vi "运维调试_采配水.vi"() -> ()   [LabVIEW 2016, in "PLC.lvlib"]
uses:
  PLC.lvlib
  control/switch.ctl
  <vilib>/Plasmionique/MB Master/MB_Master/MB_Master.lvclass
  <vilib>/Utility/miscctls.llb/LVPointTypeDef.ctl
  <vilib>/Plasmionique/MB Master/MB_Master_Serial/MB_Master_Serial.lvclass
  D:/Program Files (x86)/National Instruments/LabVIEW 2016/vi.lib/Plasmionique/MB Master/MB_Master/MB_Master.lvclass
  <vilib>/Instr/_visa.llb/VISA Configure Serial Port (Instr).vi
  <vilib>/NI/Modbus Library/API/Wrapper/Create TCP Slave.vi
  <vilib>/NI/Modbus Library/API/slave/Modbus Slave.lvclass
  <vilib>/Plasmionique/MB Master/MB Master.lvlib
  <vilib>/ptbypt/NI_PtbyPt.lvlib
  <vilib>/NI/Modbus Library/API/Wrapper/API Main.lvlib
panel:
  in  "63μm反冲洗阀":bool
  out "R34":u16
  in  "Y21":T1
  out "供水压力":dbl format="%.4f"
  out "R44":u16
  in  "Y31":T1
  out "R111":i16 caption="三级水样池润洗时间"
  in  "三级过滤系统":bool
  out "R110":i16 caption="集气时间"
  out "R104":i16 caption="三级润洗时间"
  out "R103":i16 caption="二级润洗时间"
  out "R107":i16 caption="进气时间"
  out "R43":u16
  in  "Y30":T1
  out "Registers":u16[](array[numeric])
  out "R124":i16 caption="加标回收配水时间"
  out "R42":i16
  in  "Y29":T1
  in  "更新程序":T1
  out "R122":i16 caption="二级自来水清洗时间"
  out "R121":i16 caption="一级自来水清洗时间"
  out "R120":i16 caption="过滤自来水清洗时间"
  out "清洗次数":u16
  out "当前启动泵号":u16(ring) items=["1号泵", "2号泵"]
  out "R116":i16 caption="储水时间"
  in  "R113":u16(ring) caption="水箱储水水体" items=["自来水", "水样"]
  out "R112":i16 caption="二级水样池进样超时"
  out "R31":u16
  out "R30":u16
  out "R29":u16
  out "R28":u16
  out "R27":u16
  out "R26":u16
  out "R25":u16
  out "R24":u16
  out "R23":u16
  out "R22":u16
  out "R21":u16
  out "R20":u16
  out "R19":u16
  out "R18":u16
  out "R17":u16
  out "R16":u16
  out "R15":u16
  out "R14":u16
  out "R13":u16
  out "配水压力":dbl format="%.4f"
  in  "Y18":T1
  in  "Y17":T1
  in  "Y14":T1
  in  "Y13":T1
  in  "Y1":T1
  in  "Y0":T1
  in  "Y12":T1
  in  "Y11":T1
  in  "Y10":T1
  in  "Y9":T1
  in  "Y8":T1
  in  "Y7":T1
  out "X2":bool caption="X1"
  out "采配水版本号":string
  out "R117":i16 caption="清洗频次设定"
  out "通讯故障":bool
  in  "R100":u16(ring) caption="采水泵工作模式" items=["泵1单泵单管路", "泵2单泵单管路", "潜水泵双泵双管路", "自吸泵双泵双管路"]
  out "X10":bool caption="氨氮水样池液位开关SL3"
  out "X9":bool caption="泵2过载报警_KM2"
  out "X8":bool caption="泵1过载报警_KM1"
  out "X7":bool caption="断电检测_PA"
  out "X6":bool caption="门禁开关_AS"
  out "X5":bool caption="烟雾检测_SA"
  out "X4":bool caption="浸水检测_WIA"
  out "X3":bool caption="水流开关_FS"
  out "X1":bool
  out "X0":bool caption="采样池液位开关_SL1"
  out "R109":i16 caption="外部反冲洗时间"
  out "集成报警信息":string
  out "R108":i16 caption="进样超时时间"
  out "R106":i16 caption="排液时间"
  out "R105":i16 caption="常规模式配水时间"
  out "R102":i16 caption="沉淀时间"
  out "R101":i16 caption="一级润洗时间"
  out "R2":i16
  out "R1":i16
  out "多列列表框":i32(listbox)
  in  "Y6":T1
  in  "Y5":T1
  in  "Y4":T1
  in  "Y3":T1
  in  "Y2":T1
  in  "Y16":T1
  in  "Y15":T1
  in  "返回":T1
  in  "参数设置":T1
  in  "单步启动":T1
  in  "启动":T1
  in  "停止":T1
  # "s"
  # "流程计时："
  # "s"
  # "单步计时："
  # "MPa"
  # "配水压力："
  # "MPa"
  # "供水压力："
  # "S"
  # "S"
  # "S"
  # "S"
  # "S"
  # "S"
  # "S"
  # "S"
  # "S"
  # "S"
  # "S"
  # "次"
  # "S"
  # "S"
  # "S"
  # "S"
  # "S"
  # "S"
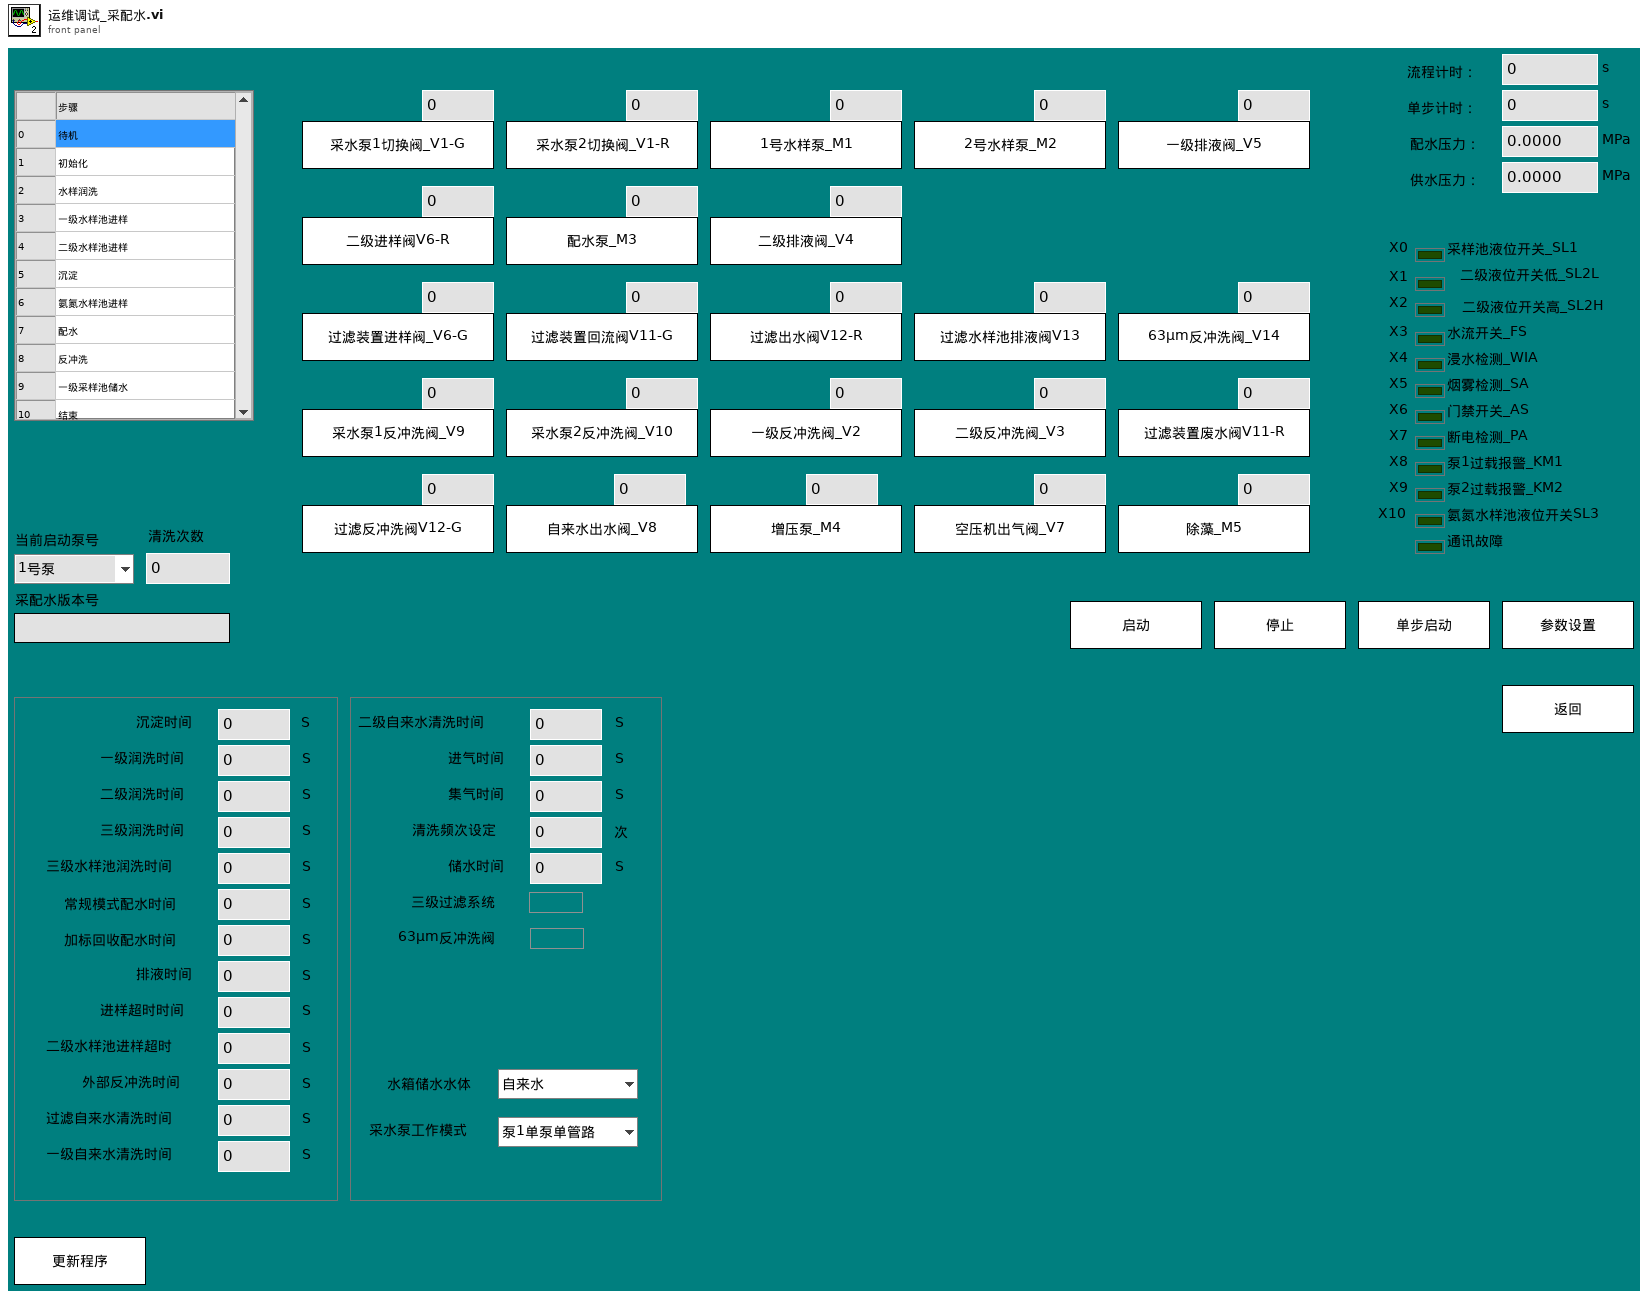
[diagram p1: front panel]
types:
  T1 = typedef "PLC.lvlib/switch.ctl" = bool
  T2 = cluster{"参数启用":cluster{"氨氮":bool, "总磷":bool, "总氮":bool, "多参数":bool, "CODMn":bool, "CODcr":bool, "超标留样":bool}}
  T3 = typedef "LVPointTypeDef.ctl" = cluster{"Horizontal":i16, "Vertical":i16}
  T4 = cluster{"状态":cluster{"R0":i16, "R1":i16, "R2":i16, "R3":i16, "R4":i16, "R5":i16, "R6":i16, "R7":i16, "R8":i16, "R9":i16, "R10":i16, "R11":i16, "R12":i16, "R13":i16, "R14":i16, "R15":i16, "R16":i16, "R17":i16, "R18":i16, "R19":i16, "R20":i16, "R21":i16, "R22":i16, "R23":i16, "R24":i16, "R25":i16, "R26":i16, "R27":i16, "R28":i16, "R29":i16, "R30":i16, "R31":i16, "R32":i16, "R33":i16, "R34":i16, "R35":i16, "R36":i16, "R37":i16, "R38":i16, "R39":i16, "R40":i16, "R41":i16, "R42":i16, "R43":i16, "R44":i16, "R45":i16, "R46":i16, "R47":i16, "R48":i16, "R49":i16, "R50":i16, "R51":i16, "R52":i16, "R53":i16, "R54":i16, "R55":i16, "R56":i16}, "输入状态":bool[], "输出状态":bool[], "参数设置":cluster{"R100":i16, "R101":i16, "R102":i16, "R103":i16, "R104":i16, "R105":i16, "R106":i16, "R107":i16, "R108":i16, "R109":i16, "R110":i16, "R111":i16, "R112":i16, "R113":i16, "R114":i16, "R115":i16, "R116":i16, "R117":i16, "R118":i16, "R119":i16, "R120":i16, "R121":i16, "R122":i16, "R123":i16, "R124":i16}, "转换值":cluster{"AD0":sgl, "AD1":sgl, "AD2":sgl, "AD3":sgl, "AD4":sgl, "AD5":sgl}}
  T5 = cluster{"R100":i16, "R101":i16, "R102":i16, "R103":i16, "R104":i16, "R105":i16, "R106":i16, "R107":i16, "R108":i16, "R109":i16, "R110":i16, "R111":i16, "R112":i16, "R113":i16, "R114":i16, "R115":i16, "R116":i16, "R117":i16, "R118":i16, "R119":i16, "R120":i16, "R121":i16, "R122":i16, "R123":i16, "R124":i16}
  T6 = cluster{"AD0":sgl, "AD1":sgl, "AD2":sgl, "AD3":sgl, "AD4":sgl, "AD5":sgl}
  T7 = cluster{"R0":i16, "R1":i16, "R2":i16, "R3":i16, "R4":i16, "R5":i16, "R6":i16, "R7":i16, "R8":i16, "R9":i16, "R10":i16, "R11":i16, "R12":i16, "R13":i16, "R14":i16, "R15":i16, "R16":i16, "R17":i16, "R18":i16, "R19":i16, "R20":i16, "R21":i16, "R22":i16, "R23":i16, "R24":i16, "R25":i16, "R26":i16, "R27":i16, "R28":i16, "R29":i16, "R30":i16, "R31":i16, "R32":i16, "R33":i16, "R34":i16, "R35":i16, "R36":i16, "R37":i16, "R38":i16, "R39":i16, "R40":i16, "R41":i16, "R42":i16, "R43":i16, "R44":i16, "R45":i16, "R46":i16, "R47":i16, "R48":i16, "R49":i16, "R50":i16, "R51":i16, "R52":i16, "R53":i16, "R54":i16, "R55":i16, "R56":i16}
  T8 = cluster{"命令":string, "数据":cluster{"starting address":u16, "holding register value":u16}}
  T9 = cluster{"时间标识":timestamp, "设备":string, "日志信息":string}
  T10 = cluster{"seconds since 1Jan1904":timestamp, "table输入":string, string, "table输入":string}
  T11 = cluster{"时间标识":timestamp, "设备":string, "日志信息":string, "流程参数":string}
  T12 = cluster{"命令":string, cluster{"starting address":u16, "holding register value":u16}}
  T13 = cluster{"命令":string, "数据":cluster{"starting address":u16, "holding register values":u16[]}}
  T14 = cluster{"命令":string, "data":cluster{"starting address":u16, "coil values":bool[]}}
  T15 = cluster{"参数启用":cluster{"氨氮":bool, "总磷总氮":bool, "总氮":bool, "多参数":bool, "CODMn":bool, "CODcr":bool, "超标留样":bool}}
  T16 = cluster{"baud rate (bps)":u32, "stop bits":u16, "parity":u16, "flow control":u16, "timeout":u32, "retries":i32}
  T17 = cluster{"starting address":u16, "holding register values":u16[]}
  T18 = cluster{"starting address":u16, "holding register value":u16}
  T19 = cluster{"starting address":u16, "coil values":bool[]}
  T20 = cluster{"Registers[0]":u16, "Registers[1]":u16, "Registers[2]":u16, "Registers[3]":u16, "Registers[4]":u16, "Registers[5]":u16, "Registers[6]":u16, "Registers[7]":u16, "Registers[8]":u16, "Registers[9]":u16, "Registers[10]":u16, "Registers[11]":u16, "Registers[12]":u16, "Registers[13]":u16, "Registers[14]":u16, "Registers[15]":u16, "Registers[16]":u16, "Registers[17]":u16, "Registers[18]":u16, "Registers[19]":u16, "Registers[20]":u16, "Registers[21]":u16, "Registers[22]":u16, "Registers[23]":u16, "Registers[24]":u16, "Registers[25]":u16, "Registers[26]":u16, "Registers[27]":u16, "Registers[28]":u16, "Registers[29]":u16, "Registers[30]":u16, "Registers[31]":u16, "Registers[32]":u16, "Registers[33]":u16, "Registers[34]":u16, "Registers[35]":u16, "Registers[36]":u16, "Registers[37]":u16, "Registers[38]":u16, "Registers[39]":u16, "Registers[40]":u16, "Registers[41]":u16, "Registers[42]":u16, "Registers[43]":u16, "Registers[44]":u16, "Registers[45]":u16, "Registers[46]":u16, "Registers[47]":u16, "Registers[48]":u16, "Registers[49]":u16, "Registers[50]":u16, "Registers[51]":u16, "Registers[52]":u16, "Registers[53]":u16, "Registers[54]":u16, "Registers[55]":u16, "Registers[56]":u16}
  T21 = cluster{"Registers[0]":u16, "Registers[1]":u16, "Registers[2]":u16, "Registers[3]":u16, "Registers[4]":u16, "Registers[5]":u16}
  T22 = cluster{"Registers[0]":u16, "Registers[1]":u16, "Registers[2]":u16, "Registers[3]":u16, "Registers[4]":u16, "Registers[5]":u16, "Registers[6]":u16, "Registers[7]":u16, "Registers[8]":u16, "Registers[9]":u16, "Registers[10]":u16, "Registers[11]":u16, "Registers[12]":u16, "Registers[13]":u16, "Registers[14]":u16, "Registers[15]":u16, "Registers[16]":u16, "Registers[17]":u16, "Registers[18]":u16, "Registers[19]":u16, "Registers[20]":u16, "Registers[21]":u16, "Registers[22]":u16, "Registers[23]":u16, "Registers[24]":u16}
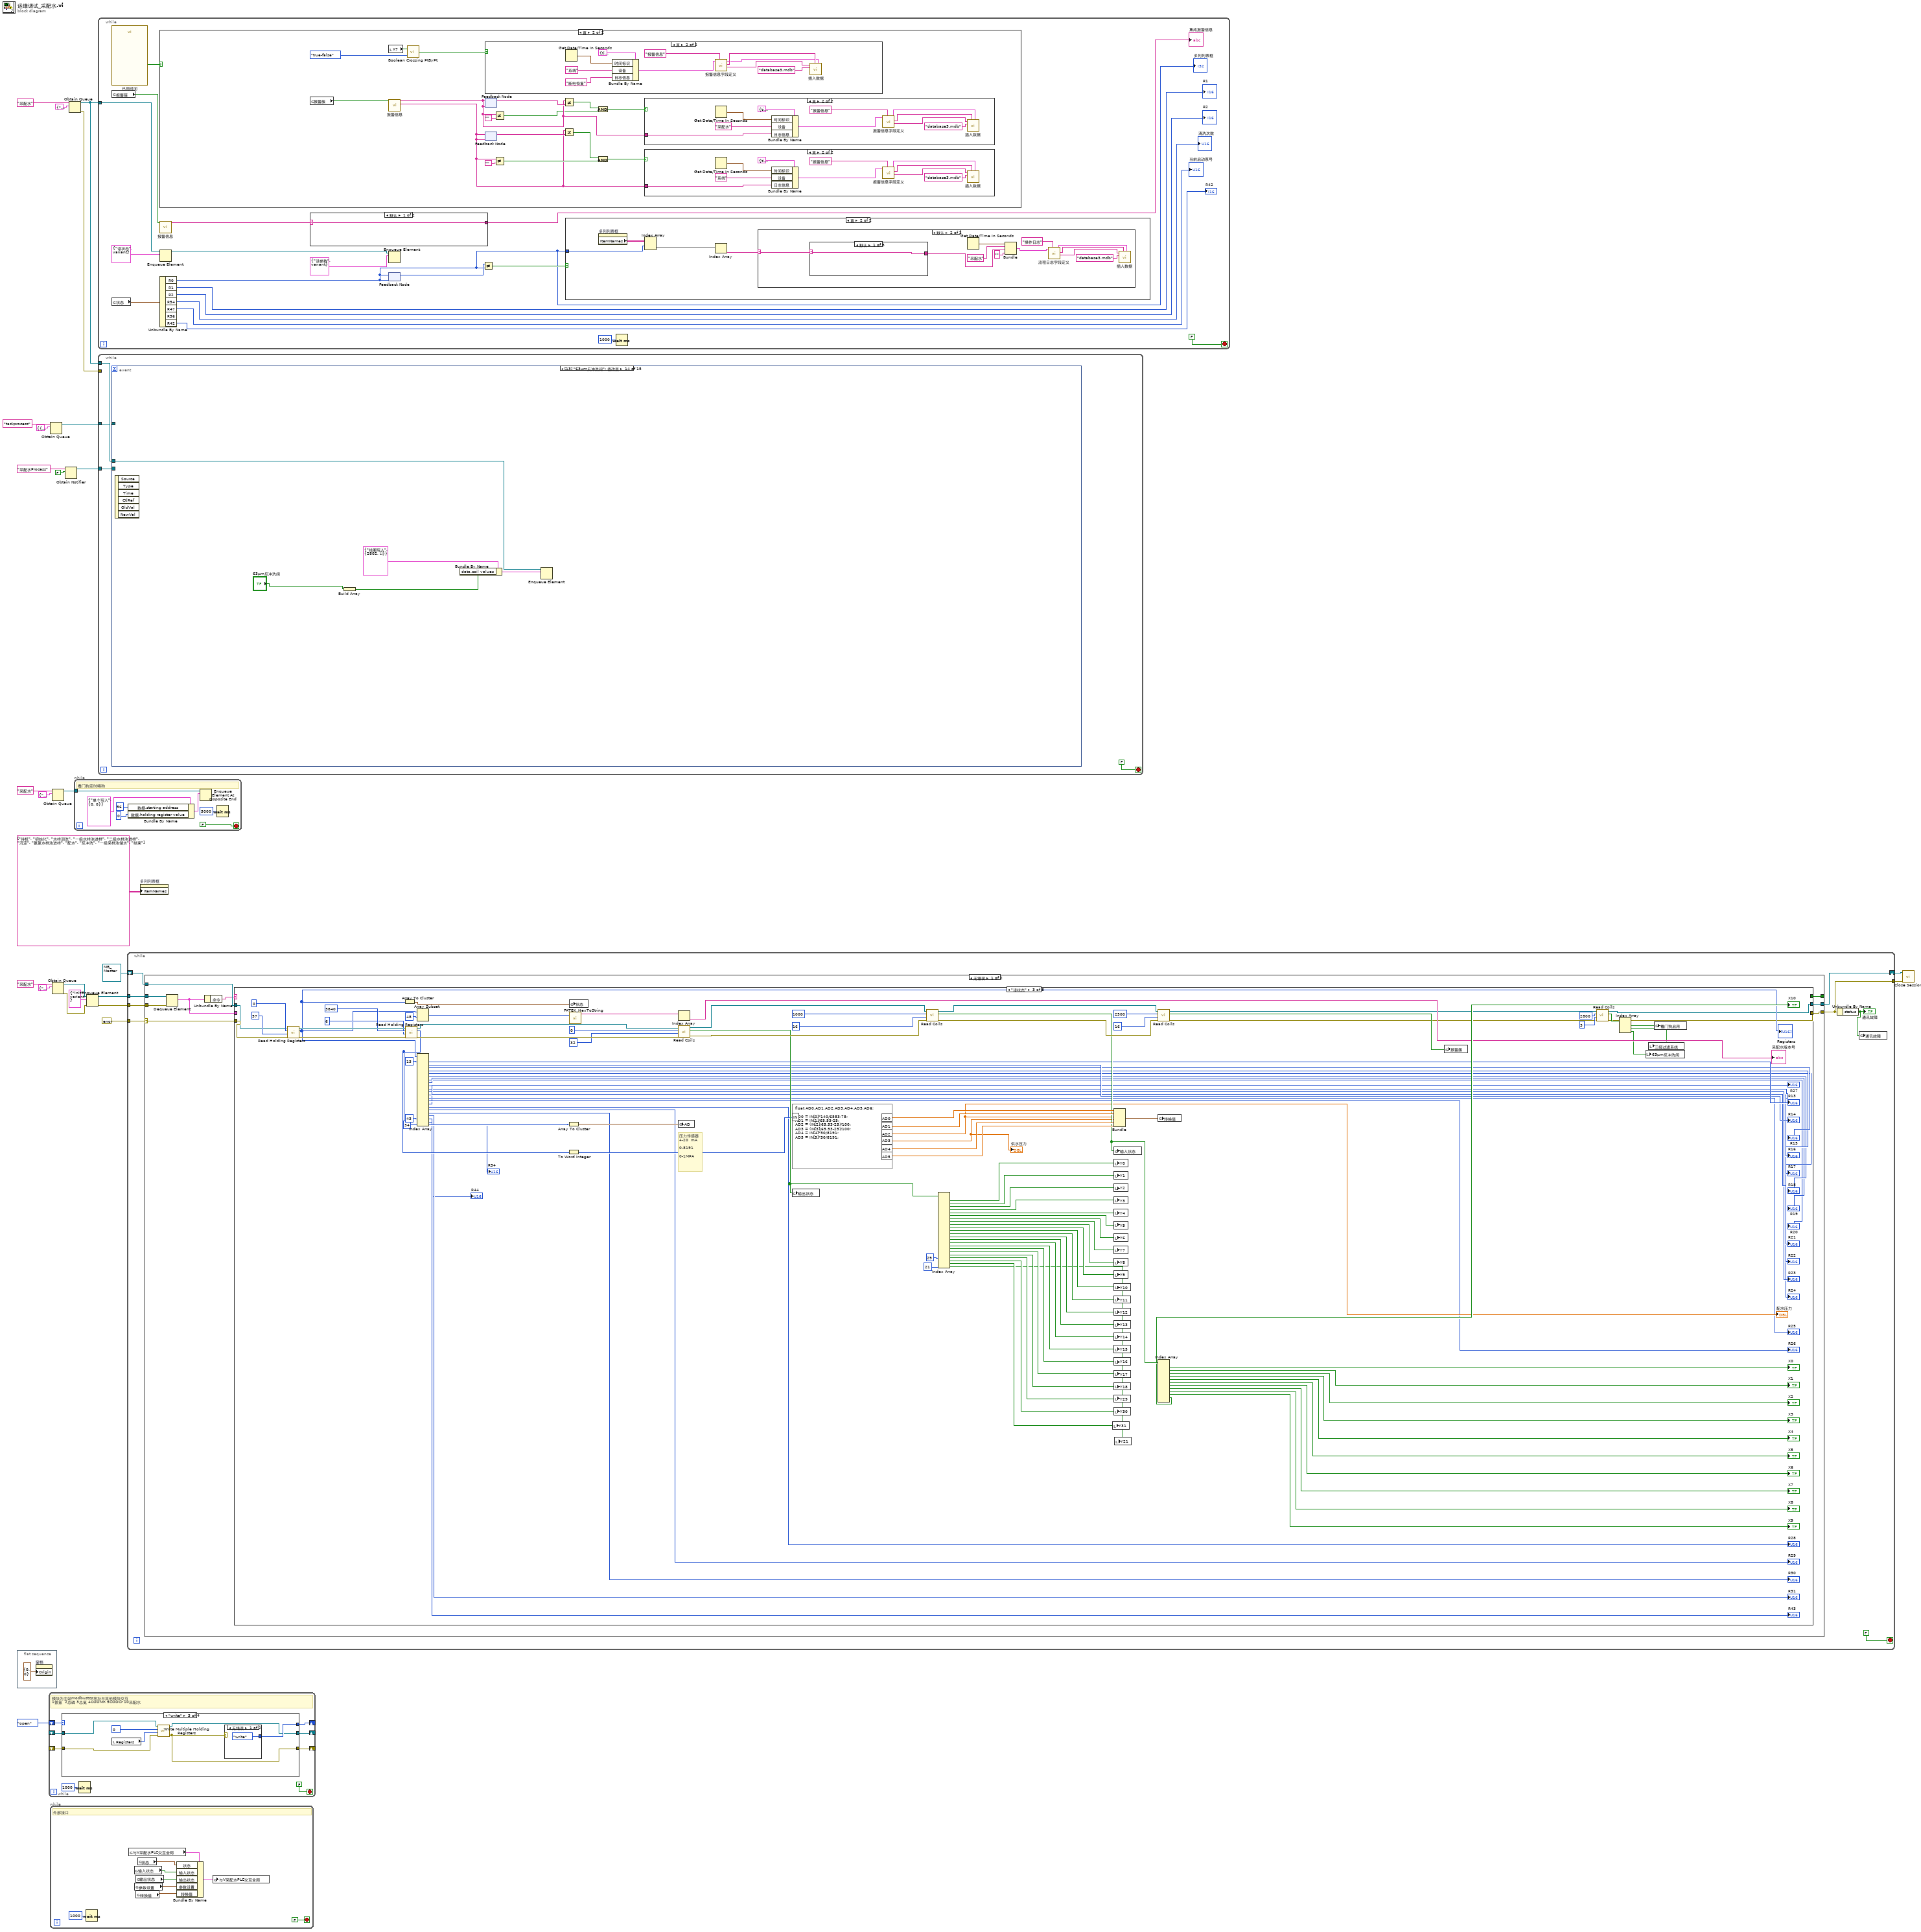
[diagram p0: block diagram]
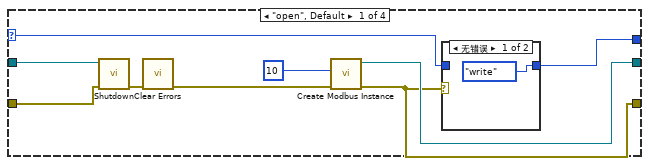
[diagram p2: hidden frame]
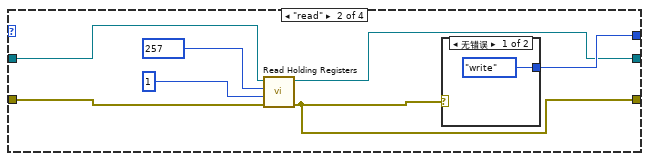
[diagram p4: hidden frame]
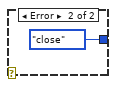
[diagram p5: hidden frame]
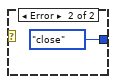
[diagram p6: hidden frame]
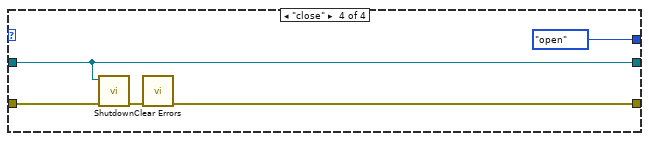
[diagram p7: hidden frame]
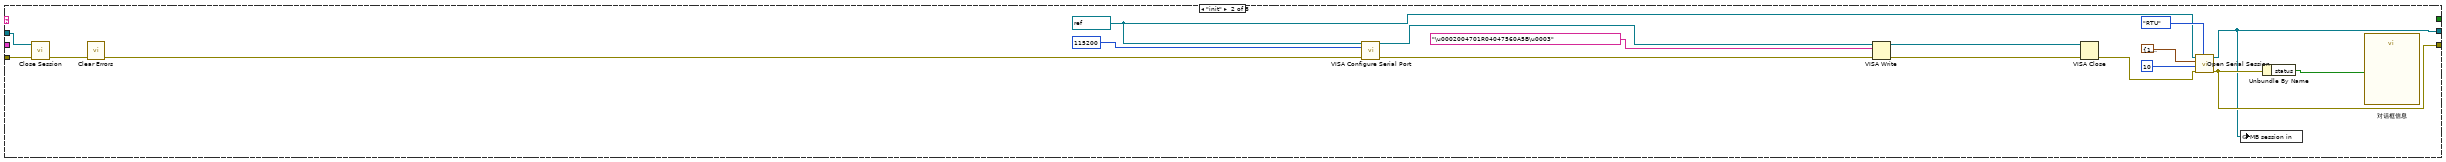
[diagram p9: hidden frame]
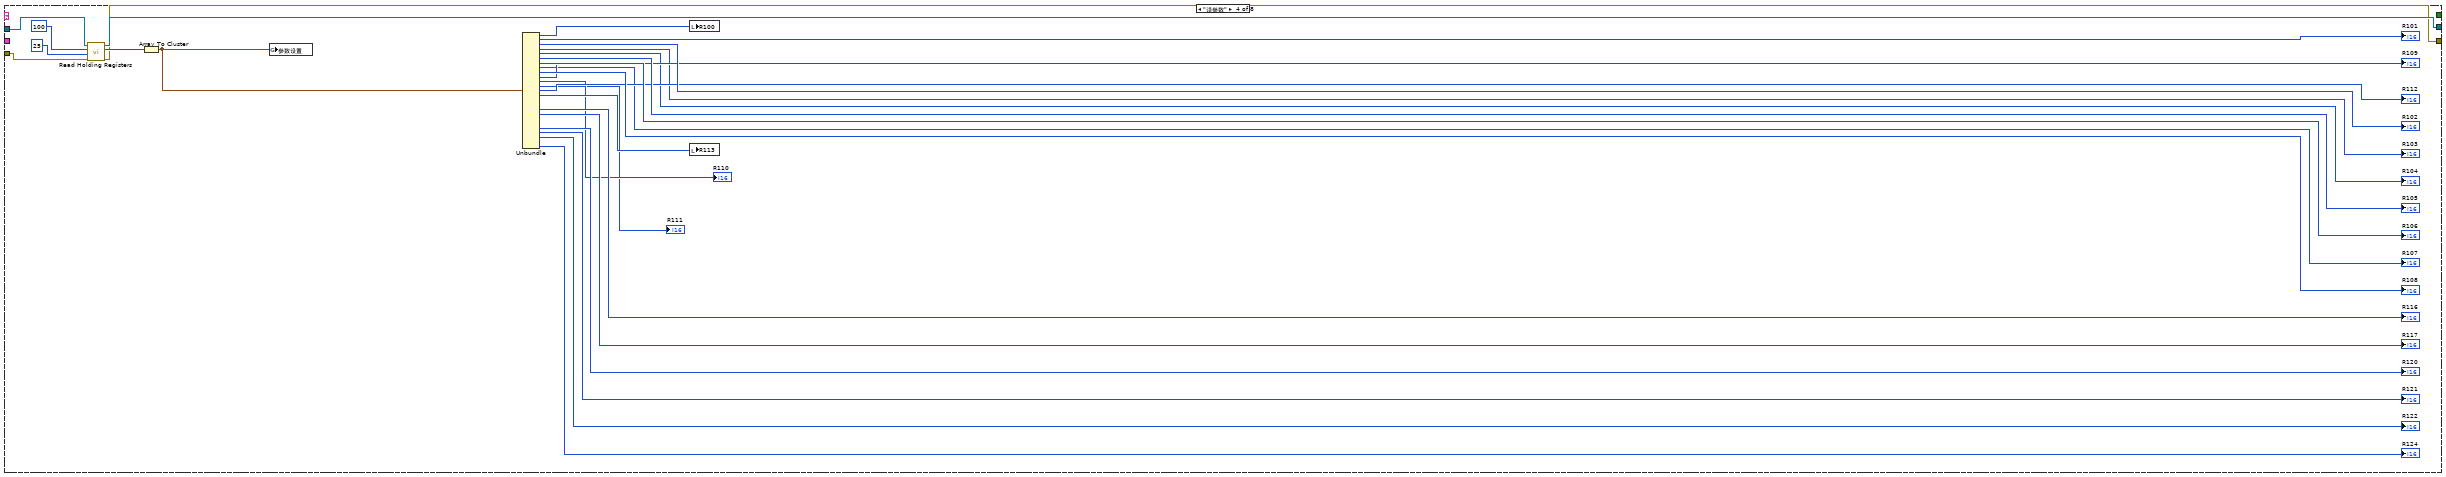
[diagram p10: hidden frame]
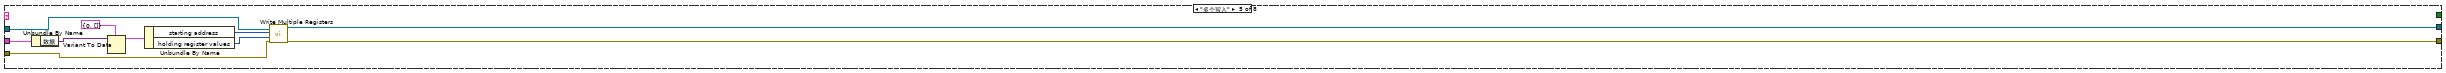
[diagram p11: hidden frame]
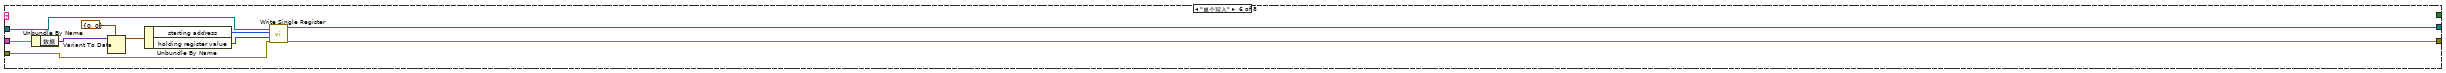
[diagram p12: hidden frame]
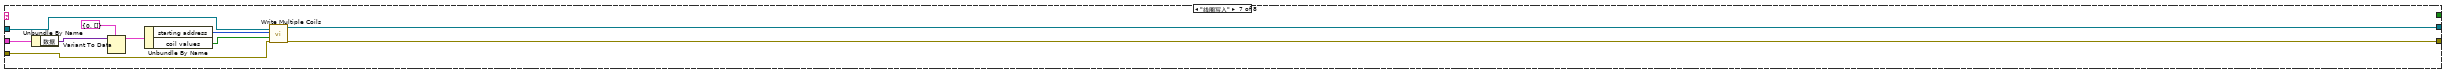
[diagram p13: hidden frame]
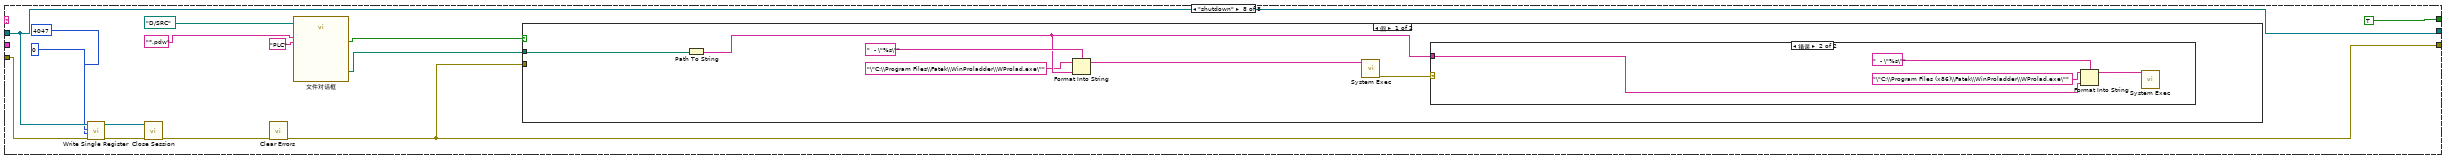
[diagram p14: hidden frame]
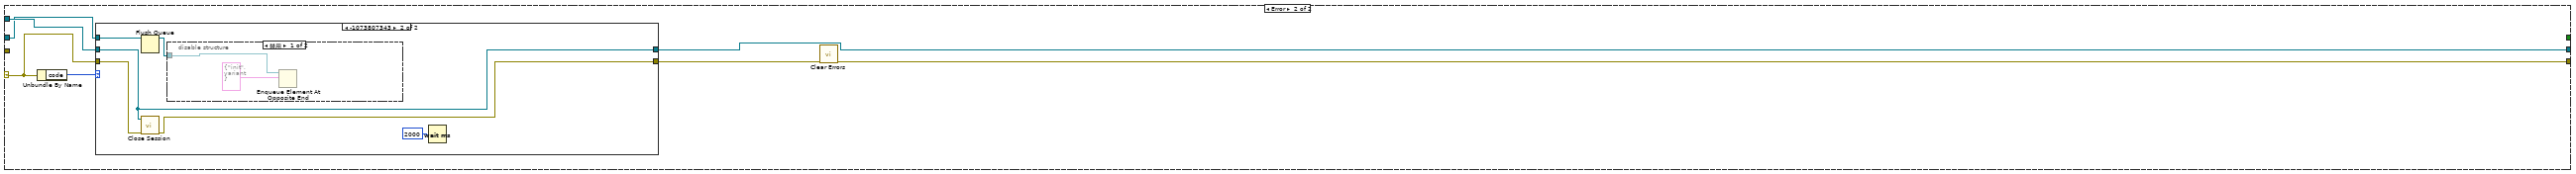
[diagram p17: hidden frame]
diagram:
  n1 = flat-sequence {
    frame #0 {
      n2 = property on="窗格" class="Pane"("Origin"=T3 {"Horizontal"=0, "Vertical"=0} ("原点")) -> ()  [unwired: 2 in, 2 out]
    }
  }
  n3 = while {
    shift-right: [w33] -> _
    shift-left: _ -> [w35]
    shift-right: [w32] -> _
    shift-left: _ -> [w34]
    shift-right: [w29] -> _
    shift-left: enum16{"open", "read", "write", "close"}."open" -> [w30]
    stop <- FALSE stop-if-true
    # "模块为主站modbustcp地址与其他模块交互\n1氨氮  2总磷 3总氮 4CODMn 5CODCr 10采配水"
    n4 = case shown="\"write\"" w30 {
      selector: w30 -> [w44 _ _ _]
      tunnel: w35 -> [w38 w50 w61 w67]
      tunnel: w34 -> [w37 w49 w58 w66]
      tunnel: [w41 w47 w57 w67] -> w33
      tunnel: [w40 w48 w56 w69] -> w32
      tunnel: [w43 w53 w62 enum16{"open", "read", "write", "close"}."open"] -> w29
      frame "open", Default {
        n5 = call-dynamic "Shutdown.vi"("error in"=w37, "Modbus slave in"=w38) -> ("error out"=w36:errorcluster)  [unwired: 9 in]
        n6 = call <vilib>:"Clear Errors.vi"("error in (no error)"=w36) -> ("error out"=w39:errorcluster)  [unwired: 5 in, 1 out]
        n7 = call-poly <vilib>:"Create Modbus Instance.vi"("error in"=w39, "port (502)"=u16 10) -> ("error out"=w40:errorcluster, "TCP slave instance"=w41:refnum<class "Modbus Slave.lvclass">)  [unwired: 8 in]
        n8 = case shown="无错误" w40 {
          tunnel: w44 -> [_ w46]
          tunnel: [enum16{"open", "read", "write", "close"}."write" w46] -> w43
          frame No Error {
          }
          frame Error {
          }
        }
      }
      frame "read" {
        n9 = call-dynamic <vilib>:"Read Holding Registers.vi"("error in"=w49, "number of inputs"=u16 1, "starting address"=u16 257, "Modbus slave in"=w50) -> ("error out"=w48:errorcluster, "Modbus slave out"=w47:refnum<class "Modbus Slave.lvclass">)  [unwired: 5 in, 1 out]
        n10 = case shown="无错误" w48 {
          tunnel: [enum16{"open", "read", "write", "close"}."write" enum16{"open", "read", "write", "close"}."close"] -> w53
          frame No Error {
          }
          frame Error {
          }
        }
      }
      frame "write" {
        n11 = local read "Registers"() -> (w59:u16[])
        n12 = call-dynamic "Write Multiple Holding Registers.vi"("error in"=w58, "registers to write"=w59, "starting address"=u16 0, "Modbus slave in"=w61) -> ("error out"=w56:errorcluster, "Modbus slave out"=w57:refnum<class "Modbus Slave.lvclass">)  [unwired: 6 in]
        n13 = case shown="无错误" w56 {
          tunnel: [enum16{"open", "read", "write", "close"}."write" enum16{"open", "read", "write", "close"}."close"] -> w62
          frame No Error {
          }
          frame Error {
          }
        }
      }
      frame "close" {
        n14 = call-dynamic "Shutdown.vi"("error in"=w66, "Modbus slave in"=w67) -> ("error out"=w65:errorcluster)  [unwired: 9 in]
        n15 = call <vilib>:"Clear Errors.vi"("error in (no error)"=w65) -> ("error out"=w69:errorcluster)  [unwired: 5 in, 1 out]
      }
    }
    n16 = Wait (ms)(milliseconds to wait=u32 1000 ("等待时间（毫秒）")) -> ()  [unwired: 1 out]
  }
  n17 = Obtain Queue(name (unnamed)="taskprocess" ("名称（未命名）"), element data type=T2 {"参数启用"={"氨氮"=FALSE, "总磷"=FALSE, "总氮"=FALSE, "多参数"=FALSE, "CODMn"=FALSE, "CODcr"=FALSE, "超标留样"=FALSE}} ("参数")) -> (queue out=w1:refnum<queue>)  [unwired: 3 in, 2 out]
  n18 = while {
    stop <- FALSE stop-if-true
    # "外部接口"
    n19 = Wait (ms)(milliseconds to wait=u32 1000 ("等待时间（毫秒）")) -> ()  [unwired: 1 out]
    n20 = global read "外部交互全局变量.vi" "与V采配水PLC交互全局"() -> (w76:T4)
    n21 = global read "采配水全局变量.vi" "输入状态"() -> (w74:bool[])
    n22 = global read "采配水全局变量.vi" "参数设置"() -> (w72:T5)
    n23 = global read "采配水全局变量.vi" "输出状态"() -> (w73:bool[])
    n24 = global read "采配水全局变量.vi" "转换值"() -> (w71:T6)
    n25 = global read "采配水全局变量.vi" "状态"() -> (w75:T7)
    n26 = Bundle By Name(cluster=w76, "状态"=w75, "输入状态"=w74, "输出状态"=w73, "参数设置"=w72, "转换值"=w71) -> (w70:T4)
    n27 = global write "外部交互全局变量.vi" "与V采配水PLC交互全局"(w70) -> ()
  }
  n28 = Obtain Queue(name (unnamed)="采配水" ("名称（未命名）"), element data type=cluster{"命令":string, "数据":variant} {"命令"="", "数据"=variant}) -> (queue out=w5:refnum<queue>)  [unwired: 3 in, 2 out]
  n29 = Obtain Queue(name (unnamed)="采配水" ("名称（未命名）"), element data type=cluster{"命令":string, "数据":variant} {"命令"="", "数据"=variant}) -> (queue out=w16:refnum<queue>, error out=w15:errorcluster)  [unwired: 3 in, 1 out]
  n30 = Obtain Notifier(name (unnamed)="采配水Process" ("名称（未命名）"), notification data type=FALSE) -> (notifier out=w19:refnum<notifier>)  [unwired: 2 in, 2 out]
  n31 = Obtain Queue(name (unnamed)="采配水" ("名称（未命名）"), element data type=cluster{"命令":string, "数据":variant} {"命令"="", "数据"=variant}) -> (queue out=w23:refnum<queue>, error out=w24:errorcluster)  [unwired: 3 in, 1 out]
  n32 = while {
    tunnel: w5 -> [w83]
    stop <- FALSE stop-if-true
    # "看门狗定时喂狗"
    n33 = Bundle By Name(cluster=T8 {"命令"="单个写入", "数据"={"starting address"=0, "holding register value"=0}} ("元素"), "数据.starting address"=u16 56, "数据.holding register value"=u16 0) -> (w84:T8)
    n34 = Enqueue Element At Opposite End(queue=w83, element=w84) -> ()  [unwired: 2 in, 3 out]
    n35 = Wait (ms)(milliseconds to wait=u32 5000 ("等待时间（毫秒）")) -> ()  [unwired: 1 out]
  }
  n36 = Enqueue Element(queue=w16, element=cluster{"命令":string, "数据":variant} {"命令"="init", "数据"=variant} ("元素"), error in (no error)=w15) -> (queue out=w11:refnum<queue>, error out=w13:errorcluster)  [unwired: 1 in, 1 out]
  n37 = while {
    tunnel: w23 -> [w103]
    stop <- FALSE stop-if-true
    n38 = call "已用时间"() -> ("Time has Elapsed"=w95:bool)  [unwired: 12 in, 7 out]
    n39 = global read "采配水全局变量.vi" "报警簇"() -> (w97:bool[])
    n40 = global read "采配水全局变量.vi" "状态"() -> (w101:T7)
    n41 = case shown="真" w95 {
      frame False {
      }
      frame True {
        n42 = global read "采配水全局变量.vi" "报警簇"() -> (w120:bool[])
        n43 = local read "X7"() -> (w107:bool)
        n44 = call "报警信息.vi"("报警簇"=w120) -> ("系统报警信息"=w109:string, "采配水报警信息"=w116:string)  [unwired: 9 in]
        n45 = call <vilib>:"Boolean Crossing PtByPt.vi"("direction"=enum16{"either", "false-true", "true-false"}."true-false", "input"=w107) -> ("crossing"=w105:bool)  [unwired: 1 in]
        n46 = case shown="真" w105 {
          frame False {
          }
          frame True {
            n47 = Get Date/Time In Seconds() -> (seconds since 1Jan1904=w129:timestamp)
            n48 = Bundle By Name(cluster=T9 {"时间标识"=timestamp(0 s since 1904-01-01), "设备"="", "日志信息"=""} ("data in"), "时间标识"=w129, "设备"="系统", "日志信息"="断电恢复") -> (w128:T9)
            n49 = call "报警信息字段定义.vi"("table输入"="报警信息", "data in"=w128) -> ("table输出"=w124:string, "columns"=w123:string[], "data out"=w122:T9)  [unwired: 7 in]
            n50 = call "插入数据.vi"("data"=w122, "columns"=w123, "database"="database3.mdb", "table"=w124) -> ()  [unwired: 7 in, 1 out]
          }
        }
        n51 = feedback #1(w116) -> (w119:string)
        n52 = feedback-in #1(w116) -> ()
        n53 = feedback #2(w109) -> (w110:string)
        n54 = feedback-in #2(w109) -> ()
        n55 = Not Equal?(x=w116, y="") -> (x != y?=w114:bool)
        n56 = Not Equal?(x=w109, y="") -> (x != y?=w113:bool)
        n57 = Not Equal?(x=w116, y=w119) -> (x != y?=w118:bool)
        n58 = Not Equal?(x=w109, y=w110) -> (x != y?=w111:bool)
        n59 = And(x=w118, y=w114) -> (x .and. y?=w117:bool)
        n60 = And(x=w111, y=w113) -> (x .and. y?=w108:bool)
        n61 = case shown="真" w117 {
          tunnel: w116 -> [_ w141]
          frame False {
          }
          frame True {
            n62 = Get Date/Time In Seconds() -> (seconds since 1Jan1904=w143:timestamp)
            n63 = Bundle By Name(cluster=T9 {"时间标识"=timestamp(0 s since 1904-01-01), "设备"="", "日志信息"=""} ("data in"), "时间标识"=w143, "设备"="采配水", "日志信息"=w141) -> (w144:T9)
            n64 = call "报警信息字段定义.vi"("table输入"="报警信息", "data in"=w144) -> ("table输出"=w148:string, "columns"=w149:string[], "data out"=w150:T9)  [unwired: 7 in]
            n65 = call "插入数据.vi"("data"=w150, "columns"=w149, "database"="database3.mdb", "table"=w148) -> ()  [unwired: 7 in, 1 out]
          }
        }
        n66 = case shown="真" w108 {
          tunnel: w109 -> [_ w131]
          frame False {
          }
          frame True {
            n67 = Get Date/Time In Seconds() -> (seconds since 1Jan1904=w133:timestamp)
            n68 = Bundle By Name(cluster=T9 {"时间标识"=timestamp(0 s since 1904-01-01), "设备"="", "日志信息"=""} ("data in"), "时间标识"=w133, "设备"="系统", "日志信息"=w131) -> (w134:T9)
            n69 = call "报警信息字段定义.vi"("table输入"="报警信息", "data in"=w134) -> ("table输出"=w138:string, "columns"=w139:string[], "data out"=w140:T9)  [unwired: 7 in]
            n70 = call "插入数据.vi"("data"=w140, "columns"=w139, "database"="database3.mdb", "table"=w138) -> ()  [unwired: 7 in, 1 out]
          }
        }
      }
    }
    n71 = call "报警信息.vi"("报警簇"=w97) -> ("采配水报警信息"=w89:string)  [unwired: 9 in, 1 out]
    n72 = Enqueue Element(queue=w103, element=cluster{"命令":string, "数据":variant} {"命令"="读状态", "数据"=variant} ("元素")) -> (queue out=w92:refnum<queue>)  [unwired: 2 in, 2 out]
    n73 = Unbundle By Name(w101) -> ("R0"=w90:i16, "R1"=→"R1":i16, "R2"=→"R2":i16, "R54"=→"清洗次数":i16, "R47"=→"当前启动泵号":i16, "R42"=→"R42":i16)  [unwired: 1 out]
    "多列列表框" <- w90
    n74 = case shown="默认" w89 {
      selector: w89 -> [w151 _]
      tunnel: [w151 w152] -> w96
      frame Default {
      }
      frame "" {
        n75 = global read "采配水全局变量.vi" "运行状态显示"() -> (w152:string)
      }
    }
    "集成报警信息" <- w96
    n76 = Enqueue Element(queue=w92, element=cluster{"命令":string, "数据":variant} {"命令"="读参数", "数据"=variant} ("元素")) -> ()  [unwired: 2 in, 3 out]
    n77 = feedback-in #3(w90) -> ()
    n78 = feedback #3(w90) -> (w91:i16)
    n79 = Not Equal?(x=w91, y=w90) -> (x != y?=w98:bool)
    n80 = case shown="真" w98 {
      tunnel: w90 -> [_ w155]
      frame False {
      }
      frame True {
        n81 = property on="多列列表框" class="MCListbox (严格)"() -> ("ItemNames"=w156:string[][])  [unwired: 2 in, 2 out]
        n82 = Index Array(array=w156, index (row)=w155) -> (element=w154:string[])  [unwired: 1 in]
        n83 = Index Array(array=w154) -> (element=w153:string)  [unwired: 1 in]
        n84 = case shown="默认" w153 {
          selector: w153 -> [_ w158]
          frame "待机" {
          }
          frame Default {
            n85 = case shown="默认" w158 {
              selector: w158 -> [w168 _ _]
              tunnel: [w168 "-->>启动" "-->>结束"] -> w157
              frame Default {
              }
              frame "初始化" {
              }
              frame "结束" {
              }
            }
            n86 = Get Date/Time In Seconds() -> (seconds since 1Jan1904=w162:timestamp)
            n87 = Bundle("seconds since 1Jan1904"=w162, "table输入"="采配水", w157, "table输入"="") -> (w160:T10)  [unwired: 1 in]
            n88 = call "流程日志字段定义.vi"("table输入"="操作日志", "data in"=w160) -> ("table输出"=w165:string, "columns"=w166:string[], "data out"=w167:T11)  [unwired: 7 in]
            n89 = call "插入数据.vi"("data"=w167, "columns"=w166, "database"="database3.mdb", "table"=w165) -> ()  [unwired: 7 in, 1 out]
          }
        }
      }
    }
    n90 = Wait (ms)(milliseconds to wait=u32 1000 ("等待时间（毫秒）")) -> ()  [unwired: 1 out]
  }
  n91 = while {
    tunnel: w23 -> [w173]
    tunnel: w24 -> [_]
    tunnel: w19 -> [w172]
    tunnel: w1 -> [w171]
    stop <- FALSE stop-if-true
    n92 = event shown="[13] \"63μm反冲洗阀\": 值改变" {
      selector: _ -> [_ _ _ _ _ _ _ _ _ _ _ _ _ _ _]
      dyn-events: _ -> [_ _ _ _ _ _ _ _ _ _ _ _ _ _ _]
      timeout: _ -> [_ _ _ _ _ _ _ _ _ _ _ _ _ _ _]
      tunnel: w173 -> [_ w178 _ w197 w216 w225 w230 _ _ _ w266 w269 w274 w279 w285]
      tunnel: w172 -> [_ w177 w182 _ _ _ _ _ _ _ _ _ _ _ _]
      tunnel: w171 -> [_ w175 w180 _ _ _ _ _ _ _ _ _ _ _ _]
      event Timeout {
        n93 = event-data() -> ()  [unwired: 1 in, 3 out]
      }
      event Value Change {
        n94 = event-data() -> ()  [unwired: 1 in, 6 out]
        n95 = Send Notification(notification=TRUE ("通知"), notifier=w177) -> ()  [unwired: 1 in, 2 out]
        n96 = Flush Queue(queue=w175) -> ()  [unwired: 1 in, 3 out]
        n97 = Enqueue Element At Opposite End(queue=w178, element=T12 {"命令"="单个写入", {"starting address"=300, "holding register value"=2}} ("元素")) -> ()  [unwired: 2 in, 3 out]
      }
      event Value Change {
        n98 = event-data() -> ()  [unwired: 1 in, 6 out]
        n99 = flat-sequence {
          tunnel: w182 -> [w184]
          tunnel: [w183] -> w181
          tunnel: w180 -> [w183]
          tunnel: w181 -> [w185]
          frame #0 {
            n100 = Cancel Notification(0:w184) -> ()  [unwired: 1 in, 3 out]
          }
          frame #1 {
            n101 = call "手动启动选择对话框.vi"() -> ("确定"=w187:bool, "输出簇"=w186:T15)  [unwired: 10 in]
            n102 = case shown="真" w187 {
              tunnel: w186 -> [_ w190]
              tunnel: w185 -> [_ w189]
              frame False {
              }
              frame True {
                n103 = global read "采配水全局变量.vi" "流程运行中"() -> (w188:bool)
                n104 = case shown="假" w188 {
                  tunnel: w190 -> [w192 _]
                  tunnel: w189 -> [w191 _]
                  frame False {
                    n105 = Enqueue Element(queue=w191, element=w192) -> ()  [unwired: 2 in, 3 out]
                  }
                  frame True {
                    n106 = One Button Dialog(message="流程已启动，无需重复启动！" ("消息")) -> ()  [unwired: 1 in, 1 out]
                  }
                }
              }
            }
          }
        }
      }
      event Value Change {
        n107 = event-data() -> ()  [unwired: 1 in, 6 out]
        n108 = call "单步启动对话框.vi"() -> ("单步启动步骤输出"=w194:u16)  [unwired: 11 in]
        n109 = Bundle By Name(cluster=T8 {"命令"="单个写入", "数据"={"starting address"=301, "holding register value"=0}} ("元素"), "数据.holding register value"=w194) -> (w195:T8)
        n110 = Enqueue Element At Opposite End(queue=w197, element=w195) -> ()  [unwired: 2 in, 3 out]
      }
      event "R101", "R102", "R105", "R106", "R108", "R109", "R100", "R112", "R113", "R103", "R104", "R107", "R110", "R111": Value Change {
        n111 = event-data() -> ()  [unwired: 1 in, 6 out]
        n112 = local read "R111"() -> (w198:i16)
        n113 = local read "R110"() -> (w199:i16)
        n114 = local read "R101"() -> (w212:i16)
        n115 = local read "R102"() -> (w211:i16)
        n116 = local read "R103"() -> (w201:i16)
        n117 = local read "R104"() -> (w200:i16)
        n118 = local read "R105"() -> (w210:i16)
        n119 = local read "R106"() -> (w209:i16)
        n120 = local read "R107"() -> (w208:i16)
        n121 = local read "R108"() -> (w207:i16)
        n122 = local read "R109"() -> (w205:i16)
        n123 = local read "R112"() -> (w203:i16)
        n124 = Build Array("R100", w212, w211, w201, w200, w210, w209, w208, w207, w205, w199, w198, w203, "R113") -> (w204:u16[])
        n125 = Bundle By Name(cluster=T13 {"命令"="多个写入", "数据"={"starting address"=0, "holding register values"=[]}} ("元素"), "数据.starting address"=u16 100, "数据.holding register values"=w204) -> (w213:T13)
        n126 = Enqueue Element At Opposite End(queue=w216, element=w213) -> ()  [unwired: 2 in, 3 out]
      }
      event "R116", "R117", "R120", "R121", "R122": Value Change {
        n127 = event-data() -> ()  [unwired: 1 in, 6 out]
        n128 = local read "R116"() -> (w223:i16)
        n129 = local read "R117"() -> (w222:i16)
        n130 = local read "R120"() -> (w221:i16)
        n131 = local read "R121"() -> (w220:i16)
        n132 = local read "R122"() -> (w219:i16)
        n133 = Build Array(w223, w222, i16 0 ("元素"), i16 0 ("R116"), w221, w220, w219) -> (w224:i16[])
        n134 = Bundle By Name(cluster=T13 {"命令"="多个写入", "数据"={"starting address"=0, "holding register values"=[]}} ("元素"), "数据.starting address"=u16 116, "数据.holding register values"=w224) -> (w226:T13)
        n135 = Enqueue Element At Opposite End(queue=w225, element=w226) -> ()  [unwired: 2 in, 3 out]
      }
      event "R124": Value Change {
        n136 = event-data() -> ("NewVal"=w229:i16)  [unwired: 1 in, 5 out]
        n137 = Build Array(w229) -> (w231:i16[])
        n138 = Bundle By Name(cluster=T13 {"命令"="多个写入", "数据"={"starting address"=0, "holding register values"=[]}} ("元素"), "数据.starting address"=u16 124, "数据.holding register values"=w231) -> (w232:T13)
        n139 = Enqueue Element At Opposite End(queue=w230, element=w232) -> ()  [unwired: 2 in, 3 out]
      }
      event "R101", "R102", "R105", "R106", "R108", "R109", "R117", "R116", "R112", "R120", "R121", "R122", "R124", "R107", "R103", "R104", "R110", "R111": Mouse Down {
        n140 = event-data() -> ("CtlRef"=w238:refnum<vi>)  [unwired: 1 in, 7 out]
        n141 = property class="DigNum (严格)"(reference=w238) -> (reference out=w236:refnum<vi>, "Value"=w237:i16)  [unwired: 1 in, 1 out]
        n142 = call "数字键盘.vi"("OldNumber"=w237) -> ("NewNumber"=w235:sgl)
        n143 = property class="DigNum (严格)"(reference=w236, "Val(Sgnl)"=w235) -> ()  [unwired: 1 in, 2 out]
      }
      event Value Change {
        n144 = event-data() -> ()  [unwired: 1 in, 6 out]
        n145 = property on="窗格" class="Pane"("Origin"=T3 {"Horizontal"=0, "Vertical"=628} ("原点")) -> ()  [unwired: 2 in, 2 out]
      }
      event Value Change {
        n146 = event-data() -> ()  [unwired: 1 in, 6 out]
        n147 = property on="窗格" class="Pane"("Origin"=T3 {"Horizontal"=0, "Vertical"=0} ("原点")) -> ()  [unwired: 2 in, 2 out]
      }
      event Value Change {
        n148 = event-data() -> ()  [unwired: 1 in, 6 out]
        n149 = Build Array("Y0", "Y1", "Y2", "Y3", "Y4", "Y5", "Y6", "Y7", "Y8", "Y9", "Y10", "Y11", "Y12", "Y13", "Y14", "Y15", "Y16", "Y17", "Y18", "Y29", "Y30", "Y31") -> (w259:T1[])
        n150 = Bundle By Name(cluster=T14 {"命令"="线圈写入", "data"={"starting address"=2400, "coil values"=[]}} ("元素"), "data.coil values"=w259) -> (w260:T14)
        n151 = Enqueue Element(queue=w266, element=w260) -> ()  [unwired: 2 in, 3 out]
      }
      event Value Change {
        n152 = event-data() -> ()  [unwired: 1 in, 6 out]
        n153 = Build Array("Y21") -> (w267:T1[])
        n154 = Bundle By Name(cluster=T14 {"命令"="线圈写入", "data"={"starting address"=2451, "coil values"=[]}} ("元素"), "data.coil values"=w267) -> (w270:T14)
        n155 = Enqueue Element(queue=w269, element=w270) -> ()  [unwired: 2 in, 3 out]
      }
      event "三级过滤系统": Value Change {
        n156 = event-data() -> ()  [unwired: 1 in, 6 out]
        n157 = Build Array("三级过滤系统") -> (w272:bool[])
        n158 = Bundle By Name(cluster=T14 {"命令"="线圈写入", "data"={"starting address"=2801, "coil values"=[]}} ("元素"), "data.coil values"=w272) -> (w275:T14)
        n159 = Enqueue Element(queue=w274, element=w275) -> ()  [unwired: 2 in, 3 out]
      }
      event "63μm反冲洗阀": Value Change {
        n160 = event-data() -> ()  [unwired: 1 in, 6 out]
        n161 = Build Array("63μm反冲洗阀") -> (w278:bool[])
        n162 = Bundle By Name(cluster=T14 {"命令"="线圈写入", "data"={"starting address"=2802, "coil values"=[]}} ("元素"), "data.coil values"=w278) -> (w280:T14)
        n163 = Enqueue Element(queue=w279, element=w280) -> ()  [unwired: 2 in, 3 out]
      }
      event Value Change {
        n164 = event-data() -> ("NewVal"=w282:T1)  [unwired: 1 in, 5 out]
        n165 = Flush Queue(queue=w285) -> (queue out=w283:refnum<queue>)  [unwired: 1 in, 2 out]
        n166 = case shown="真" w282 {
          tunnel: [cluster{"命令":string, "数据":variant} {"命令"="init", "数据"=variant} ("元素") w289] -> w284
          frame False {
          }
          frame True {
            n167 = Two Button Dialog(message="警告，非专业人士请勿进行此操作！！！\n请确认是否释放串口？" ("消息")) -> (T button?=w288:bool)  [unwired: 2 in]
            n168 = case shown="真" w288 {
              tunnel: [_ cluster{"命令":string, "数据":variant} {"命令"="shutdown", "数据"=variant} ("元素")] -> w289
              frame False {
                n169 = local write "更新程序"(FALSE ("释放串口")) -> ()
              }
              frame True {
              }
            }
          }
        }
        n170 = Enqueue Element(queue=w283, element=w284) -> ()  [unwired: 2 in, 3 out]
      }
    }
  }
  n171 = while {
    tunnel: w11 -> [w296]
    tunnel: w13 -> [w295]
    shift-right: [w299] -> w8
    shift-left: refnum<class "MB_Master.lvclass"> refnum ("MB session in") -> [w298]
    tunnel: errorcluster {"status"=FALSE, "code"=0, "source"=""} ("error out") -> [w297]
    tunnel: [w294] -> w9
    stop <- FALSE stop-if-true
    n172 = case shown="无错误" w297 {
      selector: w297 -> [w305 w525]
      tunnel: [w308 w524] -> w299
      tunnel: w298 -> [w307 w526]
      tunnel: [w306 w522] -> w294
      tunnel: w296 -> [w302 w521]
      tunnel: w295 -> [w301 _]
      tunnel: [w303 _] -> _
      frame No Error {
        n173 = Dequeue Element(queue=w302, error in (no error)=w301) -> (element=w300:cluster{"命令":string, "数据":variant})  [unwired: 1 in, 3 out]
        n174 = Unbundle By Name(w300) -> ("命令"=w304:string)
        n175 = case shown="\"读状态\"" w304 {
          tunnel: [w310 w311 w347 w461 w473 w483 w493 w508] -> w308
          tunnel: w307 -> [w310 w325 w429 w466 w476 w486 w496 w508]
          tunnel: [w309 w324 w337 w460 w474 w484 w494 w499] -> w306
          tunnel: w305 -> [w309 w327 w432 w465 w475 w485 w495 w504]
          tunnel: [_ _ _ _ _ _ _ TRUE] -> w303
          tunnel: w300 -> [_ _ _ _ w472 w482 w492 _]
          frame "idle", Default {
          }
          frame "init" {
            w315 = refnum<visa-resource-name> "COM3" ("VISA resource name")
            n176 = call-dynamic "Close Session.vi"("error in (no error)"=w327, "MB session in"=w325) -> ("error out"=w326:errorcluster)  [unwired: 9 in]
            n177 = call <vilib>:"Clear Errors.vi"("error in (no error)"=w326) -> ("error out"=w313:errorcluster)  [unwired: 5 in, 1 out]
            n178 = call-poly "VISA Configure Serial Port"("VISA resource name"=w315, "baud rate (9600)"=u32 115200, "error in (no error)"=w313) -> ("VISA resource name out"=w320:refnum<visa-resource-name>, "error out"=w319:errorcluster)  [unwired: 11 in]
            n179 = VISA Write(VISA resource name=w320, write buffer="\u0002004701R04047560A5B\u0003" ("写入缓冲区"), error in (no error)=w319) -> (VISA resource name out=w318:refnum<visa-resource-name>, error out=w317:errorcluster)  [unwired: 1 out]
            n180 = VISA Close(VISA resource name=w318, error in (no error)=w317) -> (error out=w312:errorcluster)
            n181 = call <vilib>:"Open Serial Session.vi"("Mode (RTU)"=enum16{"RTU", "ASCII"}."RTU", "Error in"=w312, "Slave ID"=u8 10, "Serial Config"=T16 {"baud rate (bps)"=115200, "stop bits"=10, "parity"=0, "flow control"=0, "timeout"=500, "retries"=1}, "VISA Resource"=w315) -> ("Error out"=w324:errorcluster, "MB_Serial session"=w311:refnum<class "MB_Master_Serial.lvclass">)  [unwired: 5 in]
            n182 = global write "采配水全局变量.vi" "MB session in"(w311) -> ()
            n183 = Unbundle By Name(w324) -> ("status"=w328:bool)
            n184 = call "对话框信息"("Enable"=w328) -> ()  [unwired: 9 in, 2 out]
          }
          frame "读状态" {
            # "压力传感器\n4-20  mA \n \n0-8191\n\n0-1MPA"
            n185 = call <vilib>:"Read Holding Registers.vi"("error in (no error)"=w432, "quantity"=u16 57 ("number of holding registers"), "starting address"=u16 0, "MB session in"=w429) -> ("error out"=w427:errorcluster, "Registers"=w372:u16[], "MB session out"=w428:refnum<class "MB_Master.lvclass">)  [unwired: 5 in]
            "Registers" <- w372
            n186 = Array To Cluster(array=w372) -> (cluster=w351:T20)
            n187 = call <vilib>:"Read Holding Registers.vi"("error in (no error)"=w427, "quantity"=u16 6 ("number of holding registers"), "starting address"=u16 3840, "MB session in"=w428) -> ("error out"=w423:errorcluster, "Registers"=w401:u16[], "MB session out"=w424:refnum<class "MB_Master.lvclass">)  [unwired: 5 in]
            n188 = Array Subset(array=w372, index=48 ("索引")) -> (w398:u16[])  [unwired: 1 in]
            n189 = Index Array(array=w372, index #1=13 ("索引"), index #20=43 ("索引"), index #22=34 ("索引")) -> (element #1=→"R13":u16, element #2=→"R14":u16, element #3=→"R15":u16, element #4=→"R16":u16, element #5=→"R17":u16, element #6=→"R18":u16, element #7=→"R19":u16, element #8=→"R20":u16, element #9=→"R21":u16, element #10=→"R22":u16, element #11=→"R23":u16, element #12=→"R24":u16, element #13=→"R25":u16, element #14=→"R26":u16, element #15=→"R27":u16, element #16=→"R28":u16, element #17=→"R29":u16, element #18=→"R30":u16, element #19=→"R31":u16, element #20=→"R43":u16, element #21=→"R44":u16, element #22=→"R34":u16)  [unwired: 19 in]
            n190 = Array To Cluster(array=w401) -> (cluster=w438:T21)
            n191 = To Word Integer(number=w401) -> (16bit integer=w400:i16[])
            n192 = global write "采配水全局变量.vi" "状态"(w351) -> ()
            n193 = call "FATEK_HexToString.vi"("数组"=w398) -> ("STRING"=w397:string[])  [unwired: 10 in]
            n194 = Index Array(array=w397) -> (element=→"采配水版本号":string)  [unwired: 1 in]
            n195 = call <vilib>:"Read Coils.vi"("error in (no error)"=w423, "quantity"=u16 32 ("number of coils"), "starting address"=u16 0, "MB session in"=w424) -> ("error out"=w419:errorcluster, "Coils"=w404:bool[], "MB session out"=w420:refnum<class "MB_Master.lvclass">)  [unwired: 5 in]
            n196 = global write "采配水全局变量.vi" "AD"(w438) -> ()
            n197 = formula code="float AD0,AD1,AD2,AD3,AD4,AD5,AD6;\n\nAD0 = IN[0]*140/6553-75;\nAD1 = IN[1]/65.53-25;\nAD2 = (IN[2]/65.53-25)/100;\nAD3 = (IN[3]/65.53-25)/100;\nAD4 = IN[4]*30/8191;\nAD5 = IN[5]*30/8191;"("IN"=w400) -> ("AD0"=w436:dbl, "AD1"=w435:dbl, "AD2"=w380:dbl, "AD3"=w334:dbl, "AD4"=w434:dbl, "AD5"=w433:dbl)
            "配水压力" <- w380
            "供水压力" <- w334
            n198 = global write "采配水全局变量.vi" "输出状态"(w404) -> ()
            n199 = call <vilib>:"Read Coils.vi"("error in (no error)"=w419, "quantity"=u16 16 ("number of coils"), "starting address"=u16 1000, "MB session in"=w420) -> ("error out"=w415:errorcluster, "Coils"=w411:bool[], "MB session out"=w416:refnum<class "MB_Master.lvclass">)  [unwired: 5 in]
            n200 = Index Array(array=w404, index #20=29 ("索引"), index #23=21 ("索引")) -> (element #1=w379:bool, element #2=w395:bool, element #3=w394:bool, element #4=w393:bool, element #5=w392:bool, element #6=w391:bool, element #7=w390:bool, element #8=w386:bool, element #9=w385:bool, element #10=w384:bool, element #11=w383:bool, element #12=w382:bool, element #13=w381:bool, element #14=w378:bool, element #15=w377:bool, element #16=w376:bool, element #17=w375:bool, element #18=w374:bool, element #19=w373:bool, element #20=w349:bool, element #21=w342:bool, element #22=w336:bool, element #23=w330:bool)  [unwired: 21 in]
            n201 = local write "Y31"(w336) -> ()
            n202 = Bundle(w436, w435, w380, w334, w434, w433) -> (w437:cluster{dbl, dbl, dbl, dbl, dbl, dbl})  [unwired: 1 in]
            n203 = global write "采配水全局变量.vi" "输入状态"(w411) -> ()
            n204 = local write "Y0"(w379) -> ()
            n205 = local write "Y1"(w395) -> ()
            n206 = local write "Y2"(w394) -> ()
            n207 = local write "Y3"(w393) -> ()
            n208 = local write "Y4"(w392) -> ()
            n209 = local write "Y5"(w391) -> ()
            n210 = local write "Y6"(w390) -> ()
            n211 = local write "Y7"(w386) -> ()
            n212 = local write "Y8"(w385) -> ()
            n213 = local write "Y9"(w384) -> ()
            n214 = local write "Y10"(w383) -> ()
            n215 = local write "Y11"(w382) -> ()
            n216 = local write "Y12"(w381) -> ()
            n217 = local write "Y13"(w378) -> ()
            n218 = local write "Y14"(w377) -> ()
            n219 = local write "Y15"(w376) -> ()
            n220 = local write "Y16"(w375) -> ()
            n221 = local write "Y17"(w374) -> ()
            n222 = local write "Y18"(w373) -> ()
            n223 = local write "Y29"(w349) -> ()
            n224 = local write "Y30"(w342) -> ()
            n225 = local write "Y21"(w330) -> ()
            n226 = call <vilib>:"Read Coils.vi"("error in (no error)"=w415, "quantity"=u16 16 ("number of coils"), "starting address"=u16 2500, "MB session in"=w416) -> ("error out"=w338:errorcluster, "Coils"=w412:bool[], "MB session out"=w348:refnum<class "MB_Master.lvclass">)  [unwired: 5 in]
            n227 = global write "采配水全局变量.vi" "转换值"(w437) -> ()
            n228 = Index Array(array=w411) -> (element #1=→"X0":bool, element #2=→"X1":bool, element #3=→"X2":bool, element #4=→"X3":bool, element #5=→"X4":bool, element #6=→"X5":bool, element #7=→"X6":bool, element #8=→"X7":bool, element #9=→"X8":bool, element #10=→"X9":bool, element #11=→"X10":bool)  [unwired: 12 in, 1 out]
            n229 = global write "采配水全局变量.vi" "报警簇"(w412) -> ()
            n230 = call <vilib>:"Read Coils.vi"("error in (no error)"=w338, "quantity"=u16 3, "starting address"=u16 2800, "MB session in"=w348) -> ("error out"=w337:errorcluster, "Coils"=w344:bool[], "MB session out"=w347:refnum<class "MB_Master.lvclass">)  [unwired: 5 in]
            n231 = Index Array(array=w344) -> (element #1=w343:bool, element #2=w339:bool, element #3=w329:bool)  [unwired: 3 in]
            n232 = local write "63μm反冲洗阀"(w329) -> ()
            n233 = local write "三级过滤系统"(w339) -> ()
            n234 = global write "采配水全局变量.vi" "看门狗启用"(w343) -> ()
          }
          frame "读参数" {
            n235 = call <vilib>:"Read Holding Registers.vi"("error in (no error)"=w465, "quantity"=u16 25 ("number of holding registers"), "starting address"=u16 100, "MB session in"=w466) -> ("error out"=w460:errorcluster, "Registers"=w462:u16[], "MB session out"=w461:refnum<class "MB_Master.lvclass">)  [unwired: 5 in]
            n236 = Array To Cluster(array=w462) -> (cluster=w453:T22)
            n237 = global write "采配水全局变量.vi" "参数设置"(w453) -> ()
            n238 = Unbundle(w453) -> ("Registers[0]"=w452:u16, "Registers[1]"=→"R101":u16, "Registers[2]"=→"R102":u16, "Registers[3]"=→"R103":u16, "Registers[4]"=→"R104":u16, "Registers[5]"=→"R105":u16, "Registers[6]"=→"R106":u16, "Registers[7]"=→"R107":u16, "Registers[8]"=→"R108":u16, "Registers[9]"=→"R109":u16, "Registers[10]"=→"R110":u16, "Registers[11]"=→"R111":u16, "Registers[12]"=→"R112":u16, "Registers[13]"=w449:u16, "Registers[16]"=→"R116":u16, "Registers[17]"=→"R117":u16, "Registers[20]"=→"R120":u16, "Registers[21]"=→"R121":u16, "Registers[22]"=→"R122":u16, "Registers[24]"=→"R124":u16)  [unwired: 5 out]
            n239 = local write "R100"(w452) -> ()
            n240 = local write "R113"(w449) -> ()
          }
          frame "多个写入" {
            n241 = Unbundle By Name(w472) -> ("数据"=w471:variant)
            n242 = Variant To Data(type=T17 {"starting address"=0, "holding register values"=[]}, Variant=w471) -> (data=w469:T17)  [unwired: 1 in, 1 out]
            n243 = Unbundle By Name(w469) -> ("starting address"=w468:u16, "holding register values"=w467:u16[])
            n244 = call <vilib>:"Write Multiple Registers.vi"("error in (no error)"=w475, "values"=w467, "starting address"=w468, "MB session in"=w476) -> ("error out"=w474:errorcluster, "MB session out"=w473:refnum<class "MB_Master.lvclass">)  [unwired: 6 in]
          }
          frame "单个写入" {
            n245 = Unbundle By Name(w482) -> ("数据"=w481:variant)
            n246 = Variant To Data(type=T18 {"starting address"=0, "holding register value"=0}, Variant=w481) -> (data=w479:T18)  [unwired: 1 in, 1 out]
            n247 = Unbundle By Name(w479) -> ("starting address"=w478:u16, "holding register value"=w477:u16)
            n248 = call <vilib>:"Write Single Register.vi"("error in (no error)"=w485, "value"=w477, "address"=w478, "MB session in"=w486) -> ("error out"=w484:errorcluster, "MB session out"=w483:refnum<class "MB_Master.lvclass">)  [unwired: 6 in]
          }
          frame "线圈写入" {
            n249 = Unbundle By Name(w492) -> ("数据"=w491:variant)
            n250 = Variant To Data(type=T19 {"starting address"=0, "coil values"=[]}, Variant=w491) -> (data=w489:T19)  [unwired: 1 in, 1 out]
            n251 = Unbundle By Name(w489) -> ("starting address"=w488:u16, "coil values"=w487:bool[])
            n252 = call <vilib>:"Write Multiple Coils.vi"("error in (no error)"=w495, "values"=w487, "starting address"=w488, "MB session in"=w496) -> ("error out"=w494:errorcluster, "MB session out"=w493:refnum<class "MB_Master.lvclass">)  [unwired: 6 in]
          }
          frame "shutdown" {
            n253 = call <vilib>:"Write Single Register.vi"("error in (no error)"=w504, "value"=u16 0, "address"=u16 4047, "MB session in"=w508) -> ("error out"=w503:errorcluster, "MB session out"=w507:refnum<class "MB_Master.lvclass">)  [unwired: 6 in]
            n254 = call-dynamic "Close Session.vi"("error in (no error)"=w503, "MB session in"=w507) -> ("error out"=w509:errorcluster)  [unwired: 9 in]
            n255 = call <vilib>:"Clear Errors.vi"("error in (no error)"=w509) -> ("error out"=w499:errorcluster)  [unwired: 5 in, 1 out]
            n256 = call "文件对话框"("start path"=path "D:/SRC", "pattern (all files)"="*.pdw", "pattern label"="PLC") -> ("selected path"=w502:path, "cancelled"=w500:bool)  [unwired: 9 in, 2 out]
            n257 = case shown="假" w500 {
              tunnel: w502 -> [w515 _]
              tunnel: w499 -> [_ _]
              frame False {
                n258 = Path To String(path=w515) -> (string=w512:string)
                n259 = Format Into String(format string="  - \"%s\"" ("格式字符串"), initial string="\"C:\\Program Files\\Fatek\\WinProladder\\WProlad.exe\"" ("command line"), w512) -> (resulting string=w513:string)  [unwired: 1 in, 1 out]
                n260 = call <vilib>:"System Exec.vi"("command line"=w513) -> ("error out"=w516:errorcluster)  [unwired: 7 in, 3 out]
                n261 = case shown="错误" w516 {
                  tunnel: w512 -> [_ w519]
                  frame No Error {
                  }
                  frame Error {
                    n262 = Format Into String(format string="  - \"%s\"" ("格式字符串"), initial string="\"C:\\Program Files (x86)\\Fatek\\WinProladder\\WProlad.exe\"" ("command line"), w519) -> (resulting string=w517:string)  [unwired: 1 in, 1 out]
                    n263 = call <vilib>:"System Exec.vi"("command line"=w517) -> ()  [unwired: 7 in, 4 out]
                  }
                }
              }
              frame True {
              }
            }
          }
        }
      }
      frame Error {
        n264 = Unbundle By Name(w525) -> ("code"=w527:i32)
        n265 = case shown="-1073807343" w527 {
          tunnel: w526 -> [w529 w533]
          tunnel: w525 -> [w528 w535]
          tunnel: [w528 w534] -> w523
          tunnel: [w529 w533] -> w524
          tunnel: w521 -> [_ w532]
          frame Default {
          }
          frame -1073807343 {
            n266 = Flush Queue(queue=w532) -> (queue out=w531:refnum<queue>)  [unwired: 1 in, 2 out]
            n267 = call-dynamic "Close Session.vi"("error in (no error)"=w535, "MB session in"=w533) -> ("error out"=w534:errorcluster)  [unwired: 9 in]
            n268 = disable-structure shown="禁用" {
              disable-tunnel: w531 -> [w536 _]
              frame Disabled {
                n269 = Enqueue Element At Opposite End(queue=w536, element=cluster{"命令":string, "数据":variant} {"命令"="init", "数据"=variant} ("元素")) -> ()  [unwired: 2 in, 3 out]
              }
              frame Enabled {
              }
            }
            n270 = Wait (ms)(milliseconds to wait=u32 2000 ("等待时间（毫秒）")) -> ()  [unwired: 1 out]
          }
        }
        n271 = call <vilib>:"Clear Errors.vi"("error in (no error)"=w523) -> ("error out"=w522:errorcluster)  [unwired: 5 in, 1 out]
      }
    }
    n272 = Unbundle By Name(w294) -> ("status"=w292:bool)
    "通讯故障" <- w292
    n273 = global write "采配水全局变量.vi" "通讯故障"(w292) -> ()
  }
  n274 = property on="多列列表框" class="MCListbox (严格)"("ItemNames"=string[][] [["待机"], ["初始化"], ["水样润洗"], ["一级水样池进样"], ["二级水样池进样"], ["沉淀"], ["氨氮水样池进样"], ["配水"], ["反冲洗"], ["一级采样池储水"], ["结束"]] ("项名")) -> ()  [unwired: 2 in, 2 out]
  n275 = call-dynamic "Close Session.vi"("error in (no error)"=w9, "MB session in"=w8) -> ()  [unwired: 9 in, 1 out]
